vi "Add Arc to Exit.vi"(8 "Additional circle arc (rad)":dbl, 9 "Tangent Point":cluster{dbl, dbl}, 10 "Radius":dbl, 11 "Center Point":cluster{dbl, dbl}) -> (1 "Point Arrays":cluster{dbl[], dbl[], dbl[]}, 3 "Blend Exit Point":cluster{dbl, dbl})   [LabVIEW 2019]
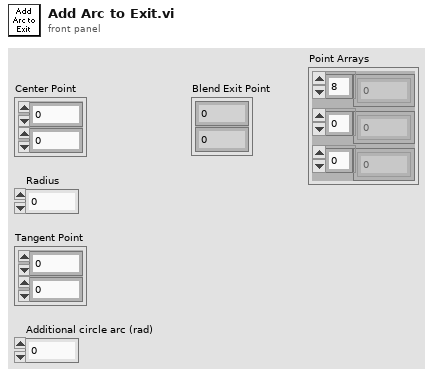
[diagram p1: front panel]
types:
  T1 = cluster{"appended array":dbl[], "appended array":dbl[], "appended array":dbl[]}
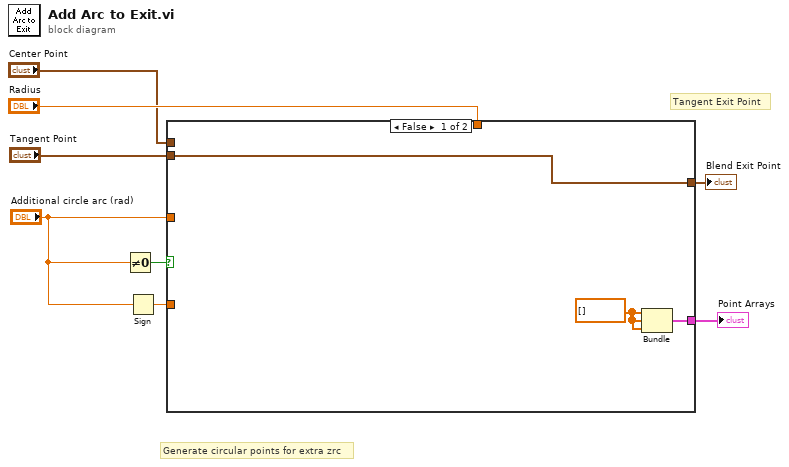
[diagram p0: block diagram]
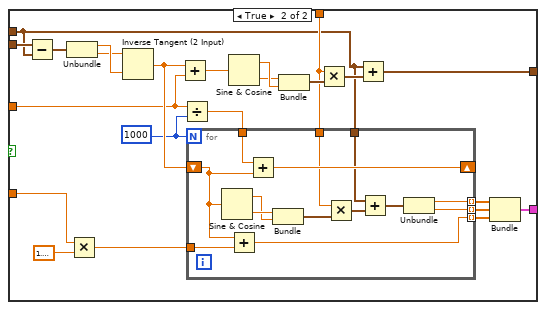
[diagram p2: hidden frame]
diagram:
  # "Generate circular points for extra zrc"
  # "Tangent Exit Point"
  n1 = Not Equal To 0?(x="Additional circle arc (rad)") -> (x != 0?=w4:bool)
  n2 = Sign(1:"Additional circle arc (rad)") -> (0:w2:dbl)
  n3 = case shown="False" w4 {
    tunnel: [w11 w34] -> w8
    tunnel: "Tangent Point" -> [w11 w26]
    tunnel: "Additional circle arc (rad)" -> [_ w23]
    tunnel: "Radius" -> [_ w20]
    tunnel: "Center Point" -> [_ w19]
    tunnel: [w10 w16] -> w3
    tunnel: w2 -> [_ w13]
    frame False {
      w9 = dbl[] [] ("appended array")
      n4 = Bundle("appended array"=w9, "appended array"=w9, "appended array"=w9) -> (w10:T1)  [unwired: 1 in]
    }
    frame True {
      w21 = 1000
      n5 = Subtract(x=w26, y=w19) -> (x-y=w27:cluster{dbl, dbl})
      n6 = Unbundle(w27) -> (w29:dbl, w28:dbl)
      n7 = Multiply(x=w13, y=1.5707963267948966) -> (x*y=w12:dbl)
      n8 = Inverse Tangent (2 Input)(1:w29, 2:w28) -> (0:w25:dbl)
      n9 = Add(x=w25, y=w23) -> (x+y=w24:dbl)
      n10 = Divide(x=w23, y=w21) -> (x/y=w22:dbl)
      n11 = for {
        N: w21 -> [_]
        shift-right: [w46] -> _
        shift-left: w25 -> [w37]
        tunnel: w22 -> [w45]
        tunnel: w19 -> [w43]
        tunnel: w20 -> [w42]
        tunnel: [w39] -> w18 mode=indexing
        tunnel: [w38] -> w17 mode=indexing
        tunnel: [w36] -> w15 mode=indexing
        tunnel: w12 -> [w35]
        n12 = Sine & Cosine(0:w37) -> (1:w47:dbl, 2:w48:dbl)
        n13 = Add(x=w37, y=w35) -> (x+y=w36:dbl)
        n14 = Add(x=w45, y=w37) -> (x+y=w46:dbl)
        n15 = Bundle(w48, w47) -> (w41:cluster{dbl, dbl})  [unwired: 1 in]
        n16 = Multiply(x=w42, y=w41) -> (x*y=w44:cluster{dbl, dbl})
        n17 = Add(x=w43, y=w44) -> (x+y=w40:cluster{dbl, dbl})
        n18 = Unbundle(w40) -> (w39:dbl, w38:dbl)
      }
      n19 = Sine & Cosine(0:w24) -> (1:w31:dbl, 2:w30:dbl)
      n20 = Bundle(w30, w31) -> (w32:cluster{dbl, dbl})  [unwired: 1 in]
      n21 = Multiply(x=w20, y=w32) -> (x*y=w33:cluster{dbl, dbl})
      n22 = Add(x=w19, y=w33) -> (x+y=w34:cluster{dbl, dbl})
      n23 = Bundle(w18, w17, w15) -> (w16:cluster{dbl[], dbl[], dbl[]})  [unwired: 1 in]
    }
  }
  "Blend Exit Point" <- w8
  "Point Arrays" <- w3
